vi "Read Integration ON.vi"(8 "error in (no error)":errorcluster, 11 "Yokogawa WT2X0 in":refnum<class "Yokogawa WT2X0.lvclass">) -> (0 "error out":errorcluster, 2 "Integration ON":bool, 3 "Yokogawa WT2X0 out":refnum<class "Yokogawa WT2X0.lvclass">)   [LabVIEW 2013, in "Universal Power Meter.lvlib" / "Yokogawa WT2X0.lvlib" / "Yokogawa WT2X0.lvclass"]
uses:
  Yokogawa WT2X0.lvclass
  Yokogawa WT2X0.lvclass/Yokogawa WT2X0.ctl
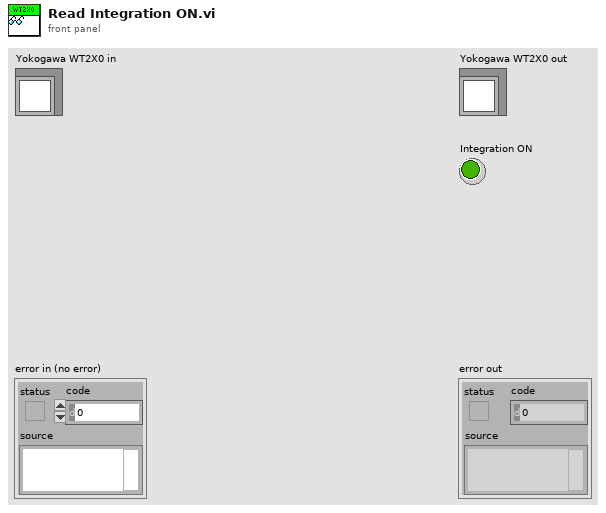
[diagram p1: front panel]
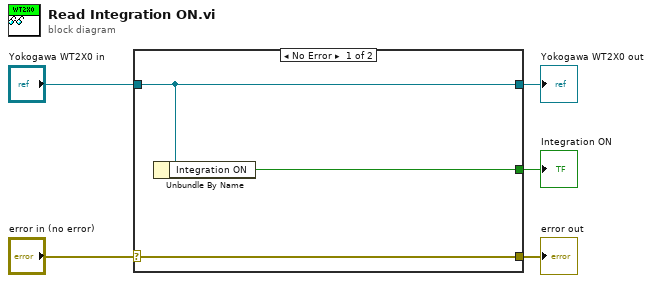
[diagram p0: block diagram]
diagram:
  n1 = case shown="No Error" "error in (no error)" {
    selector: "error in (no error)" -> [w8 w9]
    tunnel: [w8 w9] -> w4
    tunnel: [w7 w10] -> w2
    tunnel: "Yokogawa WT2X0 in" -> [w7 w10]
    tunnel: [w6 _] -> w1
    frame No Error {
      n2 = Unbundle By Name(w7) -> ("Integration ON"=w6:bool)
    }
    frame Error {
    }
  }
  "error out" <- w4
  "Yokogawa WT2X0 out" <- w2
  "Integration ON" <- w1
